vi "_AllThingsIoT.vi"   [LabVIEW 2019]
uses:
  ThingWorx/_TW_Subs/Thingworx_Write_Bool.vi
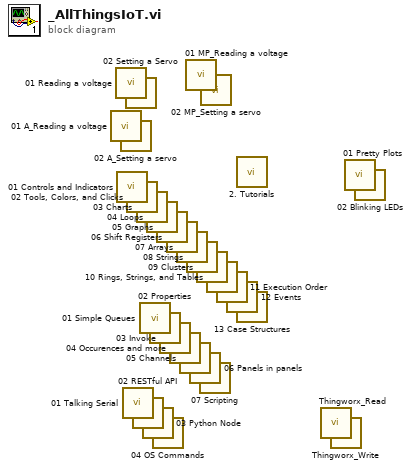
[diagram p0: block diagram]
diagram:
  n1 = call "01 A_Reading a voltage.vi"() -> ()  [unwired: 12 in]
  n2 = call "01 Reading a voltage.vi"() -> ()  [unwired: 12 in]
  n3 = call "01 Controls and Indicators.vi"() -> ()  [unwired: 12 in]
  n4 = call "02 A_Setting a servo.vi"() -> ()  [unwired: 12 in]
  n5 = call "01 Talking Serial.vi"() -> ()  [unwired: 12 in]
  n6 = call "02 Setting a Servo.vi"() -> ()  [unwired: 12 in]
  n7 = call "02 Tools, Colors, and Clicks.vi"() -> ()  [unwired: 12 in]
  n8 = call "02 RESTful API.vi"() -> ()  [unwired: 12 in]
  n9 = call "03 Charts.vi"() -> ()  [unwired: 12 in]
  n10 = call "01 Simple Queues.vi"() -> ()  [unwired: 12 in]
  n11 = call "03 Python Node.vi"() -> ()  [unwired: 12 in]
  n12 = call "04 Loops.vi"() -> ()  [unwired: 12 in]
  n13 = call "02 Properties.vi"() -> ()  [unwired: 12 in]
  n14 = call "04 OS Commands.vi"() -> ()  [unwired: 12 in]
  n15 = call "05 Graphs.vi"() -> ()  [unwired: 12 in]
  n16 = call "03 Invoke.vi"() -> ()  [unwired: 12 in]
  n17 = call "06 Shift Registers.vi"() -> ()  [unwired: 12 in]
  n18 = call "04 Occurences and more.vi"() -> ()  [unwired: 12 in]
  n19 = call "07 Arrays.vi"() -> ()  [unwired: 12 in]
  n20 = call "05 Channels.vi"() -> ()  [unwired: 12 in]
  n21 = call "01 MP_Reading a voltage.vi"() -> ()  [unwired: 12 in]
  n22 = call "08 Strings.vi"() -> ()  [unwired: 12 in]
  n23 = call "06 Panels in panels.vi"() -> ()  [unwired: 12 in]
  n24 = call "09 Clusters.vi"() -> ()  [unwired: 12 in]
  n25 = call "07 Scripting.vi"() -> ()  [unwired: 12 in]
  n26 = call "02 MP_Setting a servo.vi"() -> ()  [unwired: 12 in]
  n27 = call "10 Rings, Strings, and Tables.vi"() -> ()  [unwired: 12 in]
  n28 = call "11 Execution Order.vi"() -> ()  [unwired: 12 in]
  n29 = call "12 Events.vi"() -> ()  [unwired: 12 in]
  n30 = call "2. Tutorials.vi"() -> ()  [unwired: 12 in]
  n31 = call "13 Case Structures.vi"() -> ()  [unwired: 12 in]
  n32 = call "Thingworx_Read.vi"() -> ()  [unwired: 10 in, 2 out]
  n33 = call-poly "Thingworx_Write.vi"() -> ()  [unwired: 12 in]
  n34 = call "01 Pretty Plots.vi"() -> ()  [unwired: 12 in]
  n35 = call "02 Blinking LEDs.vi"() -> ()  [unwired: 12 in]
